vi "Query Max Voltage Limit.vi"(8 "error in (no error)":errorcluster, 9 "current limit (0.0 Amps)":dbl format="%^.2e", 10 "channel name (\"CHANNEL1\")":string="CHANNEL1", 11 "IVI_DCPwr in":refnum<class "IVI_DCPwr.lvclass">) -> (0 "error out":errorcluster, 2 "max voltage level":dbl format="%^.2e", 3 "IVI_DCPwr out":refnum<class "IVI_DCPwr.lvclass">)   [LabVIEW 2013, in "IVI_DCPwr.lvlib" / "IVI_DCPwr.lvclass"]
doc: "This VI returns the maximum programmable voltage level that the power supply accepts for a particular current limit on a channel for the output range to which the power supply is currently configured."
uses:
  IVI_DCPwr.lvclass
  IVI_DCPwr.lvclass/IVI_DCPwr.ctl
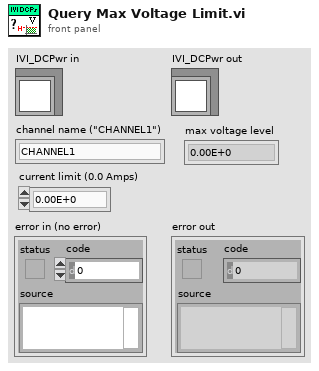
[diagram p1: front panel]
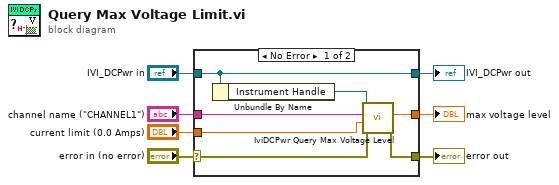
[diagram p0: block diagram]
diagram:
  n1 = case shown="No Error" "error in (no error)" {
    selector: "error in (no error)" -> [w12 w16]
    tunnel: [w11 w16] -> w6
    tunnel: [w14 w15] -> w4
    tunnel: "IVI_DCPwr in" -> [w14 w15]
    tunnel: "channel name (\"CHANNEL1\")" -> [w10 _]
    tunnel: [w9 _] -> w1
    tunnel: "current limit (0.0 Amps)" -> [w8 _]
    frame No Error {
      n2 = Unbundle By Name(w14) -> ("Instrument Handle"=w13:refnum<k15>)
      n3 = call <vilib>:"IviDCPwr Query Max Voltage Level.vi"("error in (no error)"=w12, "current limit (0.0 Amps)"=w8, "channel name (\"CHANNEL1\")"=w10, "instrument handle"=w13) -> ("error out"=w11:errorcluster, "max voltage level"=w9:dbl)  [unwired: 5 in, 1 out]
    }
    frame Error {
    }
  }
  "error out" <- w6
  "IVI_DCPwr out" <- w4
  "max voltage level" <- w1
